vi "arduino_cmd_respuesta.vi"(6 "Long":string="0", 8 "error in (no error)":errorcluster, 9 "Int":string="0", 10 "Comando":string, 11 "VISA resource name in":refnum<visa-resource-name>) -> (0 "error out":errorcluster, 2 "Respuesta":string, 3 "VISA resource name out":refnum<visa-resource-name>)   [LabVIEW 2016]
panel:
  out "Mensaje":string
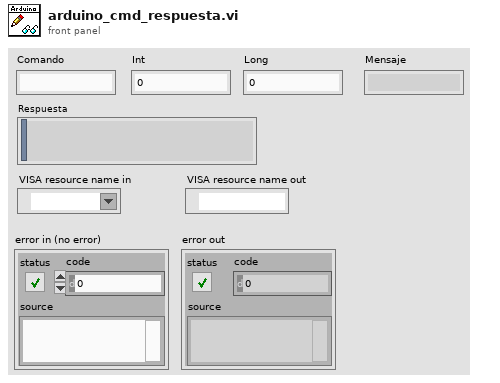
[diagram p1: front panel]
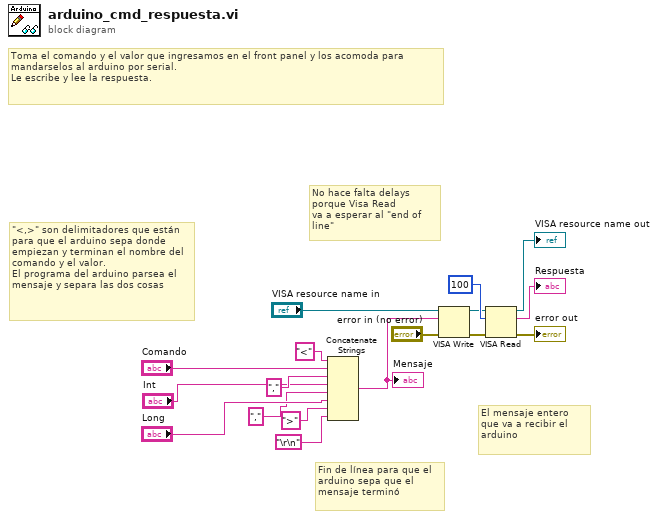
[diagram p0: block diagram]
diagram:
  # "Toma el comando y el valor que ingresamos en el front panel y los acomoda para\nmandarselos al arduino por serial.\nLe escribe y lee la respuesta."
  # "\"<,>\" son delimitadores que están\npara que el arduino sepa donde \nempiezan y terminan el nombre del comando y el valor.\nEl programa del arduino parsea el mensaje y separa las dos cosas"
  # "El mensaje entero que va a recibir el arduino"
  # "Fin de línea para que el arduino sepa que el mensaje terminó"
  # "No hace falta delays porque Visa Read\nva a esperar al \"end of line\""
  n1 = Concatenate Strings("<", "Comando", ",", "Int", ",", "Long", ">", "\r\n") -> (w11:string)
  "Mensaje" <- w11
  n2 = VISA Write(VISA resource name="VISA resource name in", write buffer=w11, error in (no error)="error in (no error)") -> (VISA resource name out=w9:refnum<visa-resource-name>, error out=w8:errorcluster)  [unwired: 1 out]
  n3 = VISA Read(VISA resource name=w9, byte count=u32 100, error in (no error)=w8) -> (VISA resource name out=→"VISA resource name out":refnum<visa-resource-name>, read buffer=→"Respuesta":string, error out=→"error out":errorcluster)  [unwired: 1 out]
